vi "get_fov.vi"(8 "error in (no error)":errorcluster, 11 "TrajectoryMH100122AODRAPS in":refnum<class "TrajectoryMH100122AODRAPS.lvclass">) -> (0 "error out":errorcluster, 1 "FOVy":dbl[unit]=0.0003, 2 "FOVx":dbl[unit]=0.0003, 3 "TrajectoryMH100122AODRAPS out":refnum<class "TrajectoryMH100122AODRAPS.lvclass">, 5 "average":dbl[unit])   [LabVIEW 2010, in "TrajectoryMH100122AODRAPS.lvclass"]
uses:
  TrajectoryMH100122AODRAPS.lvclass
  TrajectoryMH100122AODRAPS.lvclass/TrajectoryMH100122AODRAPS.ctl
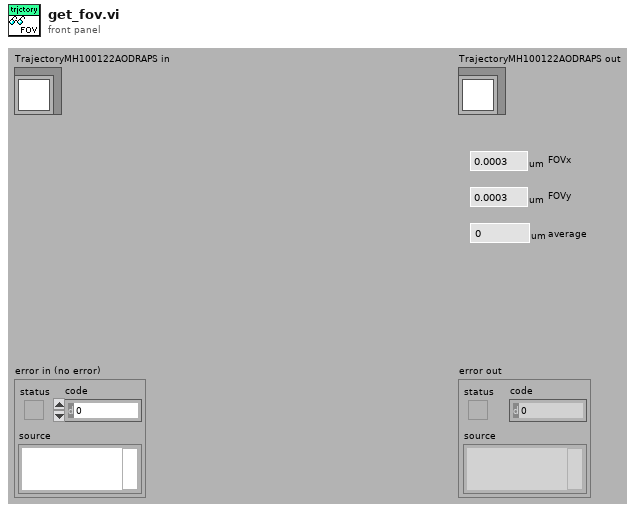
[diagram p1: front panel]
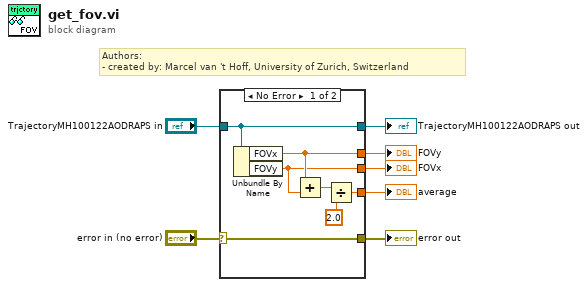
[diagram p0: block diagram]
diagram:
  # "Authors: \n- created by: Marcel van 't Hoff, University of Zurich, Switzerland"
  n1 = case shown="No Error" "error in (no error)" {
    selector: "error in (no error)" -> [w14 w16]
    tunnel: [w14 w16] -> w6
    tunnel: [w13 w15] -> w4
    tunnel: "TrajectoryMH100122AODRAPS in" -> [w13 w15]
    tunnel: [w12 _] -> w3
    tunnel: [w11 _] -> w2
    tunnel: [w8 _] -> w1
    frame No Error {
      n2 = Unbundle By Name(w13) -> ("FOVx"=w12:dbl[unit], "FOVy"=w11:dbl[unit])
      n3 = Add(x=w12, y=w11) -> (x+y=w9:dbl[unit])
      n4 = Divide(x=w9, y=2.0) -> (x/y=w8:dbl[unit])
    }
    frame Error {
    }
  }
  "error out" <- w6
  "TrajectoryMH100122AODRAPS out" <- w4
  "FOVy" <- w3
  "FOVx" <- w2
  "average" <- w1
